vi "Batch Convert USID Value for Waveforms.vi"() -> ()   [LabVIEW 2013]
panel:
  in  "Register Address":u8=28 format="%.0x"
  in  "Updated_Slave Address":u8=7
  in  "Starting Waveforms Folder":path=path "C:/Users/er080167/Documents/AD2255/Waveforms/RFFE6"
  in  "SetID Pin State":u8(ring) items=["0", "1", "Z"]
  in  "New Waveform Folder":path=path "C:/Users/er080167/Documents/AD2255/Waveforms/RFFE7"
  # "Register Address is needed to determine if .hws is extended mode"
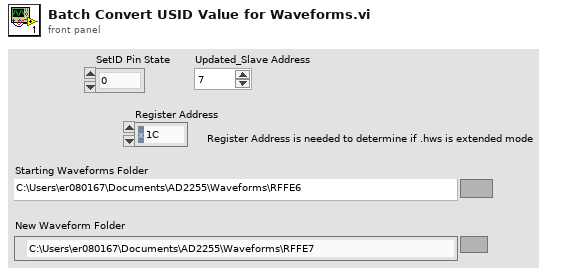
[diagram p1: front panel]
types:
  T1 = cluster{"Slave Address":u8, "Register":u8, "Data":u8}
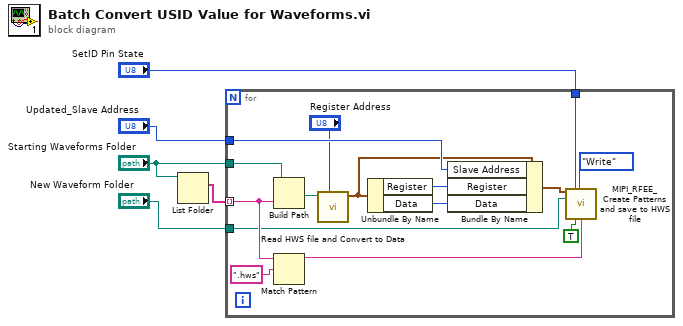
[diagram p0: block diagram]
diagram:
  n1 = List Folder(path="Starting Waveforms Folder") -> (filenames=w5:string[])  [unwired: 3 in, 3 out]
  n2 = for {
    tunnel: w5 -> [w18] mode=indexing
    tunnel: "Starting Waveforms Folder" -> [w20]
    tunnel: "New Waveform Folder" -> [w9]
    tunnel: "SetID Pin State" -> [w8]
    tunnel: "Updated_Slave Address" -> [w15]
    n3 = Build Path(base path=w20, name or relative path=w18) -> (appended path=w14:path)
    n4 = Match Pattern(string=w18, regular expression=".hws") -> (before substring=w10:string)  [unwired: 1 in, 3 out]
    n5 = call "Read HWS file and Convert to Data.vi"("Register Address"="Register Address", "Starting HWS File"=w14) -> ("Converted Data"=w13:T1)  [unwired: 9 in]
    n6 = Unbundle By Name(w13) -> ("Register"=w17:u8, "Data"=w16:u8)
    n7 = Bundle By Name(cluster=w13, "Slave Address"=w15, "Register"=w17, "Data"=w16) -> (w12:T1)
    n8 = call "MIPI_RFEE_Create Patterns and save to HWS file.vi"("Register Read/Write"=w12, "SetID Pin State"=w8, "Mode"=enum16{"Write", "Read"}."Write", "file path"=w9, "Save .HWS?"=TRUE, "Filename"=w10) -> ()  [unwired: 10 in]
  }
